vi "Mode Shift.vi"(0 "GEA2 Reference In":refnum<k24>, 5 "Standalone?":bool, 7 "Acquisition Rate (Hz)":dbl=10.0 format="%0.2f", 11 "Error In":errorcluster) -> (4 "GEA2 Reference Out":refnum<k24>, 6 "Pass/Fail?":bool, 8 "Report Text":string, 15 "Error Out":errorcluster)   [LabVIEW 2016, in "Centauro.lvlib"]
doc: "This VI performs a test to ensure the washer MC fills the tub with the appropriate amount of hot and cold water."
uses:
  Projects/Centauro.lvlib
  Q:/Common/DLLs/GEA3/GeaCommunication.dll
  Common/DLLs/GEA3/GeaCommunication.dll
  Common/LabVIEW GEA2 Toolkit/LabVIEW_GEA2_Toolkit.lvlibp/type defs/Data In.ctl
  Common/LabVIEW GEA2 Toolkit/LabVIEW_GEA2_Toolkit.lvlibp/type defs/Data Out.ctl
  <vilib>/DAQmx/write.llb/DAQmx Write (Digital 1D Bool NChan 1Samp 1Line).vi
  <vilib>/DAQmx/read.llb/DAQmx Read (Digital Wfm 1Chan NSamp).vi
  <vilib>/DAQmx/create/channels.llb/DAQmx Create Channel (DI-Digital Input).vi
  <vilib>/DAQmx/create/channels.llb/DAQmx Create Channel (DO-Digital Output).vi
  <vilib>/DAQmx/configure/timing.llb/DAQmx Timing (Sample Clock).vi
  <vilib>/DAQmx/miscellaneous.llb/DAQmx Fill In Error Info.vi
  Common/LabVIEW GEA2 Toolkit/LabVIEW_GEA2_Toolkit.lvlibp
panel:
  out "Converted Data Out":T1 {"CRC" format="%04x"; "Length" format="%02x"; "Command" format="%02x"; "Destination" format="%02x"; "Source" format="%02x"}
  in  "GEA2 Data In":T2={"Source"=228, "Destination"=33, "Command"=128, "Message"="14"} {"Command" format="%02x"; "Destination" format="%02x"; "Source" format="%02x"}
  in  "Shift to":u16(ring) items=["Spin", "Agitate"]
  in  "number of samples per channel":i32=60
  in  "9481_1 Lines":tag="9481_1/port0/line0:9481_1/port0/line3"
  in  "Modeshift Line":tag="9435_1/port0/line1"
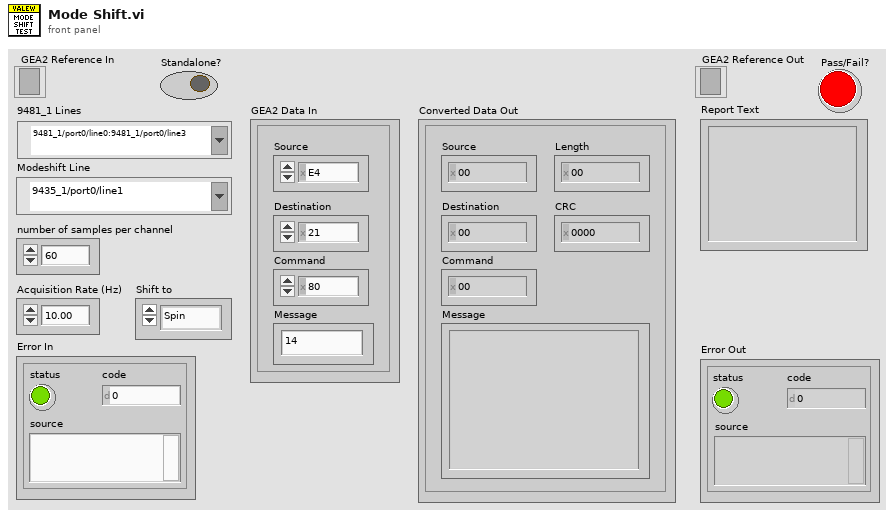
[diagram p1: front panel]
types:
  T1 = typedef "LabVIEW_GEA2_Toolkit.lvlibp/Data Out.ctl" = cluster{"Source":u8, "Destination":u8, "Command":u8, "Length":u8, "CRC":u16, "Message":string}
  T2 = typedef "LabVIEW_GEA2_Toolkit.lvlibp/Data In.ctl" = cluster{"Source":u8, "Destination":u8, "Command":u8, "Message":string}
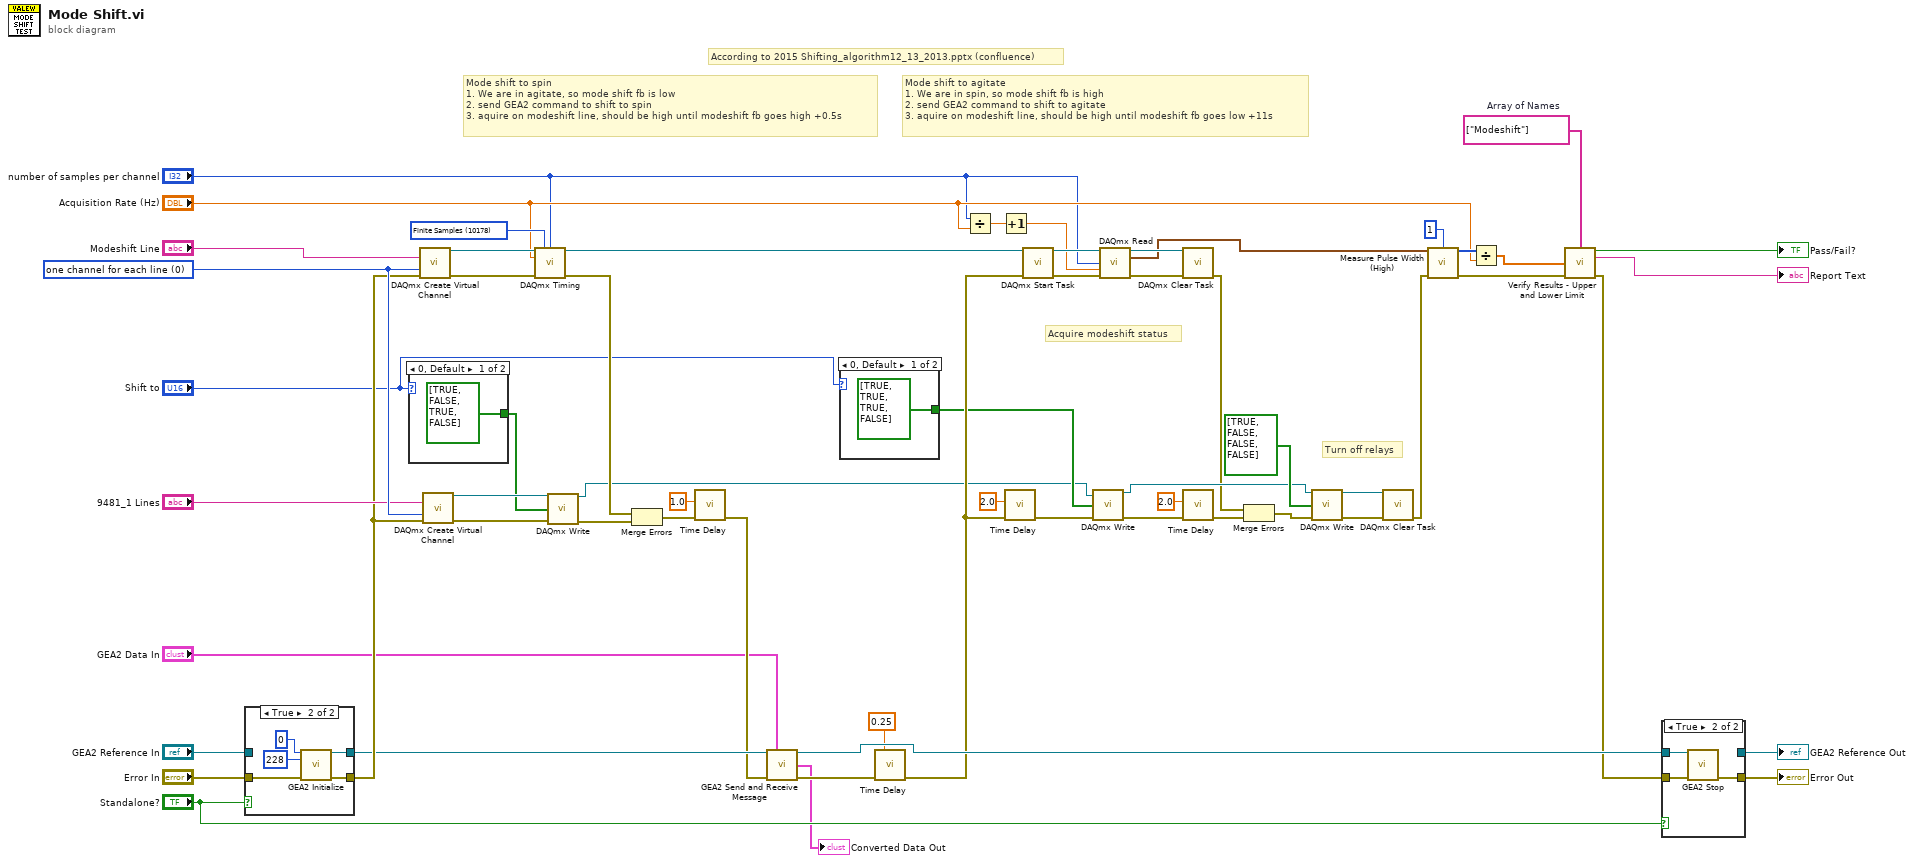
[diagram p0: block diagram]
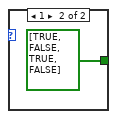
[diagram p2: hidden frame]
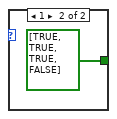
[diagram p3: hidden frame]
diagram:
  w31 = string[] ["Modeshift"]  # Array of Names
  w45 = 0 items=["one channel for each line", "one channel for all lines"] ("line grouping")
  w50 = 10178 items=["Finite Samples"=10178, "Continuous Samples"=10123, "Hardware Timed Single Point"=12522] ("sample mode")
  # "According to 2015 Shifting_algorithm12_13_2013.pptx (confluence)"
  # "Mode shift to agitate\n1. We are in spin, so mode shift fb is high\n2. send GEA2 command to shift to agitate\n3. aquire on modeshift line, should be high until modeshift fb goes low +11s"
  # "Mode shift to spin\n1. We are in agitate, so mode shift fb is low\n2. send GEA2 command to shift to spin\n3. aquire on modeshift line, should be high until modeshift fb goes high +0.5s"
  # "Turn off relays"
  # "Acquire modeshift status"
  n1 = case shown="True" "Standalone?" {
    tunnel: "Error In" -> [w62 w65]
    tunnel: [w61 w64] -> w28
    tunnel: [w62 w63] -> w40
    tunnel: "GEA2 Reference In" -> [w61 _]
    frame False {
    }
    frame True {
      n2 = call "GEA2 Initialize.vi"("Board Index"=0, "Source Address"=u8 228, "error in"=w65) -> ("GEA2 Reference Out"=w64:refnum<k24>, "error out"=w63:errorcluster)  [unwired: 10 in, 1 out]
    }
  }
  n3 = case shown="0, Default" "Shift to" {
    tunnel: [bool[] [TRUE, FALSE, TRUE, FALSE] ("data") bool[] [TRUE, TRUE, TRUE, FALSE] ("data")] -> w58
    frame 0, Default {
    }
    frame 1 {
    }
  }
  n4 = call-poly <vilib>:"DAQmx Create Virtual Channel.vi"("lines"="Modeshift Line", "line grouping"=w45, "error in"=w40) -> ("task out"=w53:refnum<k21>, "error out"=w52:errorcluster)  [unwired: 11 in]
  n5 = call-poly <vilib>:"DAQmx Create Virtual Channel.vi"("lines"="9481_1 Lines", "line grouping"=w45, "error in"=w40) -> ("task out"=w60:refnum<k21>, "error out"=w44:errorcluster)  [unwired: 11 in]
  n6 = call-poly <vilib>:"DAQmx Timing.vi"("task/channels in"=w53, "sample mode"=w50, "samples per channel"="number of samples per channel", "rate"="Acquisition Rate (Hz)", "error in"=w52) -> ("task out"=w51:refnum<k21>, "error out"=w38:errorcluster)  [unwired: 9 in]
  n7 = call-poly <vilib>:"DAQmx Write.vi"("task/channels in"=w60, "data"=w58, "error in"=w44) -> ("task out"=w18:refnum<k21>, "error out"=w39:errorcluster)  [unwired: 10 in, 1 out]
  n8 = Merge Errors(w38, w39) -> (w27:errorcluster)
  n9 = call "Time Delay"("error in (no error)"=w27, "Delay Time (s)"=1.0) -> ("error out"=w24:errorcluster)  [unwired: 9 in]
  n10 = call "GEA2 Send and Receive Message.vi"("GEA2 Reference In"=w28, "Input Data"="GEA2 Data In", "Error In"=w24) -> ("GEA2 Reference Out"=w29:refnum<k24>, "Converted Data Out"=→"Converted Data Out":T1, "Error Out"=w3:errorcluster)  [unwired: 9 in, 1 out]
  n11 = case shown="0, Default" "Shift to" {
    tunnel: [bool[] [TRUE, TRUE, TRUE, FALSE] ("data") bool[] [TRUE, FALSE, TRUE, FALSE] ("data")] -> w22
    frame 0, Default {
    }
    frame 1 {
    }
  }
  n12 = call "Time Delay"("error in (no error)"=w3, "Delay Time (s)"=0.25) -> ("error out"=w23:errorcluster)  [unwired: 9 in]
  n13 = Divide(x="number of samples per channel", y="Acquisition Rate (Hz)") -> (x/y=w11:dbl)
  n14 = Increment(x=w11) -> (x+1=w36:dbl)
  n15 = call "Time Delay"("error in (no error)"=w23, "Delay Time (s)"=2.0) -> ("error out"=w19:errorcluster)  [unwired: 9 in]
  n16 = call <vilib>:"DAQmx Start Task.vi"("task/channels in"=w51, "error in"=w23) -> ("task out"=w54:refnum<k21>, "error out"=w55:errorcluster)  [unwired: 12 in]
  n17 = call-poly <vilib>:"DAQmx Write.vi"("task/channels in"=w18, "data"=w22, "error in"=w19) -> ("task out"=w17:refnum<k21>, "error out"=w20:errorcluster)  [unwired: 10 in, 1 out]
  n18 = call-poly <vilib>:"DAQmx Read.vi"("task/channels in"=w54, "number of samples per channel"="number of samples per channel", "timeout"=w36, "error in"=w55) -> ("task out"=w57:refnum<k21>, "data"=w42:digitalwaveform, "error out"=w56:errorcluster)  [unwired: 9 in]
  n19 = call <vilib>:"DAQmx Clear Task.vi"("task in"=w57, "error in"=w56) -> ("error out"=w8:errorcluster)  [unwired: 13 in]
  n20 = call "Time Delay"("error in (no error)"=w20, "Delay Time (s)"=2.0) -> ("error out"=w7:errorcluster)  [unwired: 9 in]
  n21 = Merge Errors(w8, w7) -> (w9:errorcluster)
  n22 = call-poly <vilib>:"DAQmx Write.vi"("task/channels in"=w17, "data"=bool[] [TRUE, FALSE, FALSE, FALSE], "error in"=w9) -> ("task out"=w30:refnum<k21>, "error out"=w16:errorcluster)  [unwired: 10 in, 1 out]
  n23 = call <vilib>:"DAQmx Clear Task.vi"("task in"=w30, "error in"=w16) -> ("error out"=w6:errorcluster)  [unwired: 13 in]
  n24 = call "Measure Pulse Width (High).vi"("Input Waveform"=w42, "Minimum Pulse Width"=1, "Error In"=w6) -> ("High Iterations"=w32:i32[], "Error Out"=w33:errorcluster)  [unwired: 11 in]
  n25 = Divide(x=w32, y="Acquisition Rate (Hz)") -> (x/y=w14:dbl[])
  n26 = call "Verify Results - Upper and Lower Limit.vi"("Array of Names"=w31, "Results"=w14, "Error In"=w33) -> ("Pass/Fail?"=→"Pass/Fail?":bool, "Report Text"=→"Report Text":string, "Error Out"=w5:errorcluster)  [unwired: 9 in, 1 out]
  n27 = case shown="True" "Standalone?" {
    tunnel: w5 -> [w73 w76]
    tunnel: [w73 w75] -> w48
    tunnel: w29 -> [w72 w74]
    tunnel: [w72 _] -> w41
    frame False {
    }
    frame True {
      n28 = call "GEA2 Stop.vi"("GEA2 Reference In"=w74, "Error In"=w76) -> ("Error Out"=w75:errorcluster)  [unwired: 13 in]
    }
  }
  "Error Out" <- w48
  "GEA2 Reference Out" <- w41
